vi "Make Igor Labels.vi"(1 "Column Names":string[](array[string]), 2 "File Name":string="Test.001") -> (0 "Igor Column Headings":string)   [LabVIEW 2020]
doc: "This VI takes an input array of column names and outputs a single string of appropriately spaced column names in a format that Igor will accept for automatically nameing the columns. The file index number is appended to each column name to keep sequential data files separate\nScott Hannahs, NHMFL-FSU, February 1995"
uses:
  <vilib>/regexp/Match Regular Expression.xnode
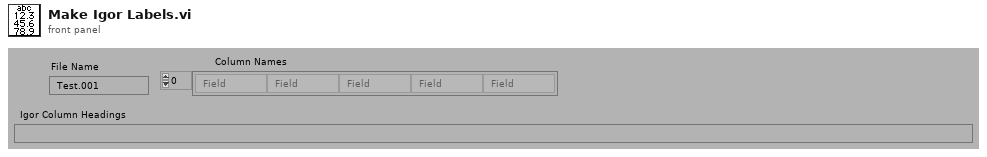
[diagram p1: front panel]
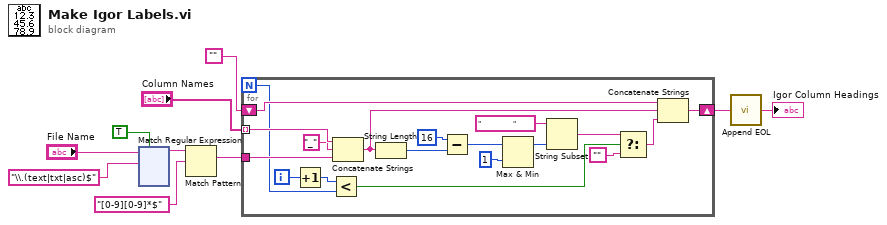
[diagram p0: block diagram]
diagram:
  n1 = xnode "Match Regular Expression"("input string"="File Name", "regular expression"="\\.(text|txt|asc)$", "ignore case? (F)"=TRUE) -> ("before match"=w1:string)  [unwired: 3 in, 4 out]
  n2 = Match Pattern(string=w1, regular expression="[0-9][0-9]*$") -> (match substring=w5:string)  [unwired: 1 in, 3 out]
  n3 = for {
    N -> [w16]
    tunnel: "Column Names" -> [w29] mode=indexing
    shift-right: [w25] -> w9
    shift-left: "" -> [w26]
    tunnel: w5 -> [w27]
    i -> [w17]
    n4 = Increment(x=w17) -> (x+1=w15:i32)
    n5 = Less?(x=w15, y=w16) -> (x < y?=w14:bool)
    n6 = Concatenate Strings(w29, "_", w27) -> (w24:string)
    n7 = String Length(string=w24) -> (length=w22:i32)
    n8 = Subtract(x=16, y=w22) -> (x-y=w19:i32)
    n9 = Max & Min(x=w19, y=1) -> (max(x,y)=w20:i32)  [unwired: 1 out]
    n10 = String Subset(string="                ", length (rest)=w20) -> (substring=w12:string)  [unwired: 1 in]
    n11 = Select(t=w12, s=w14, f="") -> (s? t:f=w13:string)
    n12 = Concatenate Strings(w26, w24, w13) -> (w25:string)
  }
  n13 = call "Append EOL.vi"("INPUT STRING"=w9) -> ("OUTPUT STRING (PLUS End of Line)"=→"Igor Column Headings":string)
